vi "ReactionWheel RT - autotuned.vi"() -> ()   [LabVIEW 2021]
uses:
  <vilib>/Platform/TimedLoop/XDataNode/timing_clust.ctl
  <vilib>/Platform/TimedLoop/XDataNode/nitl_modes.ctl
  <vilib>/Platform/TimedLoop/XDataNode/wakeup.ctl
  <vilib>/myRIO/Instrument Drivers/Onboard IO/UART/typedef/VISA Configuration.ctl
  <vilib>/myRIO/Instrument Drivers/Onboard IO/PWM/typedefs/PWM Reference.ctl
  <vilib>/myRIO/Common/Instrument Driver Framework/Utilities/typedefs/myRIO Generic Hardware Reference.ctl
  <vilib>/myRIO/Common/Instrument Driver Framework/Utilities/typedefs/Hardware Version Enum.ctl
  <vilib>/myRIO/Common/Instrument Driver Framework/Utilities/typedefs/myRIO v1.0 Reference.ctl
  <vilib>/myRIO/Common/Instrument Driver Framework/Utilities/typedefs/Generic FPGA Reference.ctl
  <vilib>/myRIO/Common/Instrument Driver Framework/myRIO v1.0/PWM/typedefs/PWM Channels Enum.ctl
  <vilib>/myRIO/Instrument Drivers/Onboard IO/PWM/typedefs/PWM Configuration.ctl
  <vilib>/userdefined/High Color/nirio_resource_hc.ctl
  <vilib>/myRIO/Common/Instrument Driver Framework/Utilities/vis/Is FPGA Ref Available.vi
  <vilib>/myRIO/Common/Instrument Driver Framework/myRIO v1.0/PWM/vis/myRIO v1.1 Open PWM.vi
  <vilib>/myRIO/Instrument Drivers/Onboard IO/PWM/vis/Set Duty Cycle and Frequency.vi
  <vilib>/myRIO/Common/Instrument Driver Framework/Utilities/vis/Validate Channels.vi
  <vilib>/myRIO/Common/Instrument Driver Framework/myRIO v1.0/PWM/vis/myRIO v1.0 Reserve PWM.vi
  <vilib>/myRIO/Common/Instrument Driver Framework/myRIO v1.0/PWM/vis/myRIO v1.0 Build MUX Configuration PWM.vi
  <vilib>/myRIO/Common/Instrument Driver Framework/myRIO v1.0/Resource Manager/vis/myRIO v1.0 Reserve Channel List.vi
  <vilib>/myRIO/Common/Instrument Driver Framework/myRIO v1.0/Resource Manager/vis/myRIO v1.0 Create Configuration List.vi
  <vilib>/myRIO/Common/Instrument Driver Framework/myRIO v1.0/Resource Manager/vis/myRIO v1.0 Reserve Channel.vi
  <vilib>/myRIO/Common/Instrument Driver Framework/myRIO v1.0/Resource Manager/vis/myRIO v1.0 Unreserve Channel.vi
  <vilib>/myRIO/Common/Instrument Driver Framework/myRIO v1.0/Resource Manager/vis/myRIO v1.0 Build Mutex Name.vi
  <vilib>/Instr/_visa.llb/VISA Configure Serial Port (Instr).vi
  <vilib>/Utility/VariantDataType/GetNumericInfo.vi
  <vilib>/Utility/error.llb/Error Cluster From Error Code.vi
  <vilib>/myRIO/Common/Instrument Driver Framework/myRIO v1.0/myRIO v1.1 Open.vi
  <vilib>/myRIO/Common/Instrument Driver Framework/Utilities/vis/IO Manager.vi
  <vilib>/myRIO/Common/Instrument Driver Framework/Utilities/vis/Configuration Manager.vi
  <vilib>/myRIO/Common/Instrument Driver Framework/myRIO v1.0/Resource Manager/vis/myRIO v1.0 Configure IO.vi
  <vilib>/myRIO/Common/Instrument Driver Framework/myRIO v1.0/myRIO v1.0 Close.vi
  <vilib>/myRIO/Common/Instrument Driver Framework/myRIO v1.0/PWM/vis/myRIO v1.0 Write PWM.vi
  <vilib>/platform/TimedLoop/XDataNode/XDataNode.xnode
  <vilib>/myRIO/Express VI/Onboard IO/UART/UART Express VI.xnode
  <vilib>/myRIO/Express VI/Onboard IO/PWM/PWM Express VI.xnode
  <vilib>/myRIO/Instrument Drivers/Onboard IO/PWM/vis/myRIO PWM Open.xnode
  <vilib>/myRIO/Instrument Drivers/Onboard IO/UART/UART.lvlib
  <vilib>/myRIO/Instrument Drivers/Onboard IO/PWM/PWM.lvlib
  <vilib>/Platform/TimedLoop/XDataNode/XDNodeRunTimeDep.lvlib
  <vilib>/addons/control/pid/NI_PID_autopid.lvlib
panel:
  in  "PID":bool
  in  "Autotune":bool
  out "Tuned PID gains":cluster{"P":dbl, "I":dbl, "D":dbl}
  in  "Deadzone off/on":bool
  out "Characters Read":string
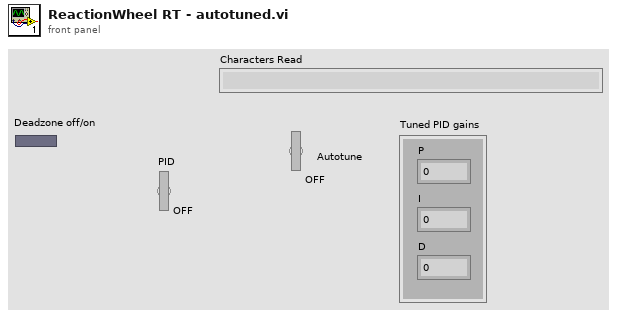
[diagram p1: front panel]
types:
  T1 = typedef "UART.lvlib/VISA Configuration.ctl" = cluster{"baud rate (9600)":u32, "data bits (8)":u16, "parity (0:none)":enum16{"None", "Odd", "Even", "Mark", "Space"}, "stop bits (10: 1 bit)":u16, "flow control (0:none)":u16, "termination char\n(0xA = '\\n' = LF) ":u8, "Enable Termination\nChar (T)":bool, "timeout (10sec)":u32}
  T2 = typedef "XDNodeRunTimeDep.lvlib/timing_clust.ctl" = cluster{"Expected End [f-1]":u64, "Actual End [f-1]":u64, "Finished Late? [f-1]":bool, "Expected End [i-1]":u64, "Actual End [i-1]":u64, "Finished Late? [i-1]":bool, "Expected Start [i]":u64, "Actual Start [i]":u64, "Expected Start [f]":u64, "Actual Start [f]":u64, "Source Name":string, "Structure Name":string, "Period":i64, "Deadline":i64, "Offset":i64, "Start":i64, "Priority":i32, "Timeout":i32, "Mode":T3, "Wakeup Reason":T4, "Error":errorcluster, "Source Type":string, "Secondary Source Type":string, "Global End Time":u64, "Global Start Time":u64, "Frame Duration":u64, "Iteration Duration":u64, "Assigned CPU":i32, "I/O Scan Engine Mode":u32}
  T3 = typedef "XDNodeRunTimeDep.lvlib/nitl_modes.ctl" = enum32{"No Change", "Process missed periods, maintain original phase", "Discard missed periods, maintain original phase", "Process missed periods, ignore original phase", "Discard missed periods, ignore original phase"}
  T4 = typedef "XDNodeRunTimeDep.lvlib/wakeup.ctl" = enum32{"Normal", "Aborted", "Asynchronous wakeup", "Timing source error", "Timed loop error", "Timeout"}
  T5 = typedef "PWM.lvlib/PWM Reference.ctl" = cluster{"myRIO Reference":T6, "PWM Channels Enum":T10, "PWM Configuration":T11}
  T6 = typedef "myRIO Generic Hardware Reference.ctl" = cluster{"myRIO Model":T7, "myRIO Hardware Reference":T8}
  T7 = typedef "Hardware Version Enum.ctl" = enum16{"Unknown", "myRIO-1900", "myRIO-1950", "roboRIO", "NI ELVIS RIO CM", "ELVIS III"}
  T8 = typedef "myRIO v1.0 Reference.ctl" = cluster{"Generic FPGA Reference":T9, "Allow multiple opens":bool}
  T9 = typedef "Generic FPGA Reference.ctl" = refnum<k20>
  T10 = typedef "PWM Channels Enum.ctl" = enum16{"Not Connected", "C/PWM0", "C/PWM1", "A/PWM0", "A/PWM1", "A/PWM2", "A/PWM3", "A/PWM4", "A/PWM5", "A/PWM6", "A/PWM7", "A/PWM8", "A/PWM9", "A/PWM10", "A/PWM11", "A/PWM12", "A/PWM13", "A/PWM14", "A/PWM15", "A/PWM16", "A/PWM17", "A/PWM18", "A/PWM19", "B/PWM0", "B/PWM1", "B/PWM2", "B/PWM3", "B/PWM4", "B/PWM5", "B/PWM6", "B/PWM7", "B/PWM8", "B/PWM9", "B/PWM10", "B/PWM11", "B/PWM12", "B/PWM13", "B/PWM14", "B/PWM15", "B/PWM16", "B/PWM17", "B/PWM18", "B/PWM19", "PWM/PWM0", "PWM/PWM1", "PWM/PWM2", "PWM/PWM3", "PWM/PWM4", "PWM/PWM5", "PWM/PWM6", "PWM/PWM7", "PWM/PWM8", "PWM/PWM9"}
  T11 = typedef "PWM.lvlib/PWM Configuration.ctl" = cluster{"Frequency":dbl, "Duty Cycle":dbl}
  T12 = typedef "nirio_resource_hc.ctl" = tag
  T13 = cluster{"proportional gain (Kc)":dbl, "integral time (Ti, min)":dbl, "derivative time (Td, min)":dbl}
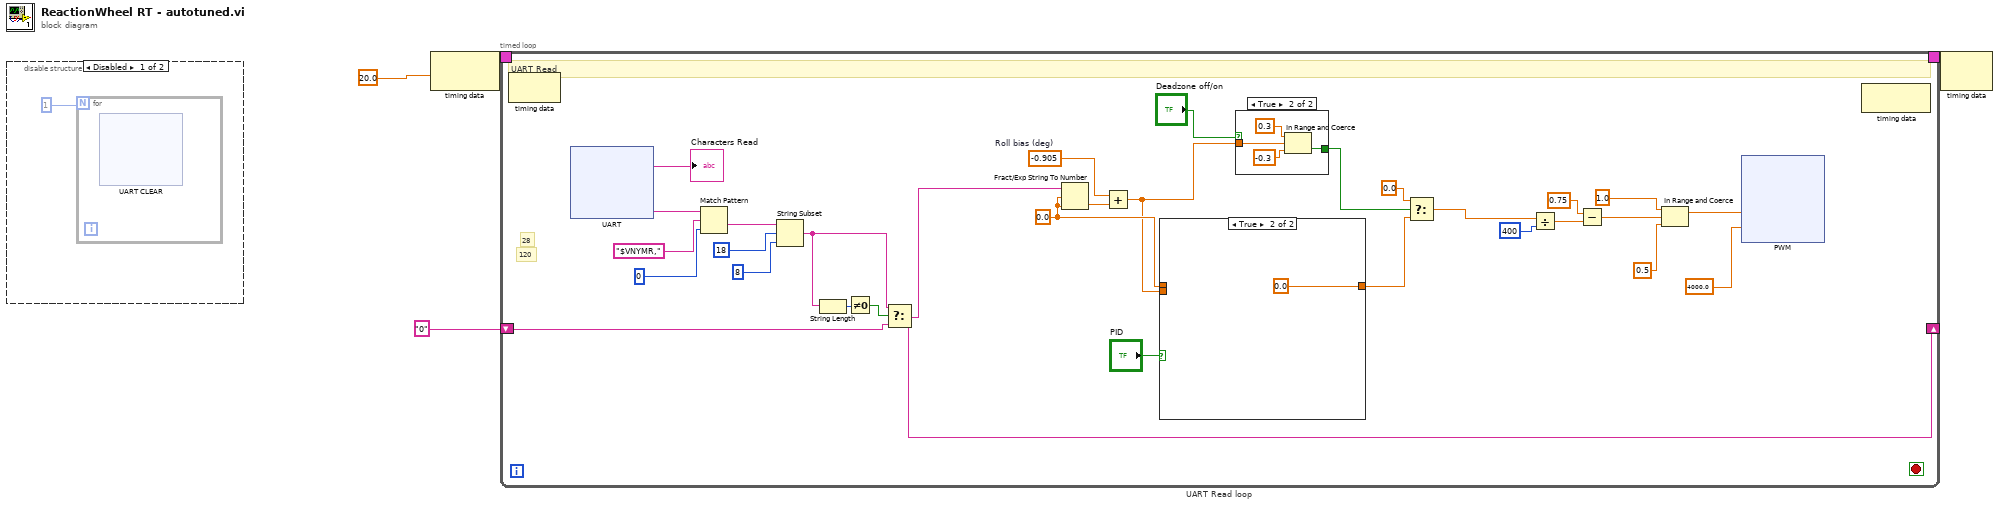
[diagram p0: block diagram]
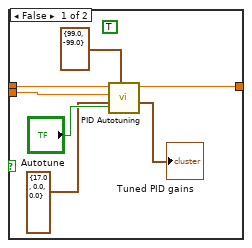
[diagram p2: hidden frame]
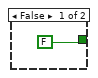
[diagram p3: hidden frame]
diagram:
  n1 = disable-structure shown="Disabled" {
    frame Disabled {
      n2 = for {
        N: 1 -> [_]
        n3 = xnode "UART CLEAR"() -> ()  [unwired: 1 in, 2 out]
      }
    }
    frame Enabled {
    }
  }
  n4 = node-c288(20.0 ("UART read period (ms)")) -> (w4:T2)
  n5 = timed-loop "UART Read loop" {
    timing: w4 -> [_]
    timing-out: [_] -> w3
    shift-right: [w31] -> _
    shift-left: "0" -> [w32]
    stop <- _ stop-if-true
    w44 = -0.905  # Roll bias (deg)
    w25 = 0.0
    # "28"
    # "120"
    # "UART Read"
    n6 = node-c288() -> ()  [unwired: 1 in, 1 out]
    n7 = xnode "UART"() -> ("Characters Read"=w51:string)  [unwired: 1 in, 1 out]
    "Characters Read" <- w51
    n8 = Match Pattern(string=w51, regular expression="$VNYMR,", offset (0)=0) -> (after substring=w50:string)  [unwired: 3 out]
    n9 = String Subset(string=w50, offset (0)=18, length (rest)=8) -> (substring=w33:string)
    n10 = String Length(string=w33) -> (length=w35:i32)
    n11 = Not Equal To 0?(x=w35) -> (x != 0?=w34:bool)
    n12 = Select(t=w33, s=w34, f=w32) -> (s? t:f=w31:string)
    n13 = Fract/Exp String To Number(string=w31, offset=w25, default (0 dbl)=w25) -> (number=w45:dbl)  [unwired: 1 in, 1 out]
    n14 = Add(x=w44, y=w45) -> (x+y=w24:dbl)
    n15 = case shown="True" "PID" {
      tunnel: w25 -> [w58 _]
      tunnel: w24 -> [w55 _]
      tunnel: [w52 0.0] -> w26
      frame False {
        (unwired) TRUE
        n16 = call <vilib>:"PID Autotuning.vi"("autotune? (F)"="Autotune", "output range"=cluster{"Maximum":dbl, "Minimum":dbl} {"Maximum"=99.0, "Minimum"=-99.0} ("PID output range"), "PID gains"=cluster{"P":dbl, "I":dbl, "D":dbl} {"P"=17.0, "I"=0.0, "D"=0.0}, "process variable"=w55, "setpoint"=w58) -> ("PID gains out"=→"Tuned PID gains":T13, "output"=w52:dbl)  [unwired: 3 in, 2 out]
      }
      frame True {
      }
    }
    n17 = case shown="True" "Deadzone off/on" {
      tunnel: [FALSE w64] -> w29
      tunnel: w24 -> [_ w63]
      frame False {
      }
      frame True {
        n18 = In Range and Coerce(upper limit=0.3 ("Angle deadzone upper limit"), x=w63, lower limit=-0.3 ("Angle deadzone lower limit")) -> (In Range?=w64:bool)  [unwired: 1 out]
      }
    }
    n19 = Select(t=0.0, s=w29, f=w26) -> (s? t:f=w30:dbl)
    n20 = Divide(x=w30, y=400) -> (x/y=w36:dbl)
    n21 = Subtract(x=0.75, y=w36) -> (x-y=w41:dbl)
    n22 = In Range and Coerce(upper limit=1.0 ("Max PWM"), x=w41, lower limit=0.5 ("Min PWM")) -> (coerced(x)=w42:dbl)  [unwired: 1 out]
    n23 = xnode "PWM"("Duty Cycle"=w42, "Frequency [Hz]"=4000.0 ("PWMfrekvens")) -> ()  [unwired: 1 in, 1 out]
    n24 = node-c288() -> ()  [unwired: 1 in, 1 out]
  }
  n25 = node-c288(w3) -> ()  [unwired: 1 out]
